vi "HTS_WAIT_FOR_READY.vi"(8 "Error IN":errorcluster, 10 "Polling time(ms)":u32=100, 11 "VISA resource IN":refnum<visa-resource-name>="COM1") -> (0 "Error OUT":errorcluster, 1 "READY?":bool=TRUE, 2 "RESPONSE":string[](array[string])=["SYSTEM STATUS: ", "0x0", "2 PUMPS", "PUMP_1 STATUS: ", "0x60", "PUMP_2 STATUS: ", "0x60", "AXIS X STATUS: ", "0x9", "AXIS Y STATUS: ", "0x9", "AXIS P STATUS: ", "0x9", "AXIS Z STATUS: ", "0x9", "NO ERROR, READY", ">"], 3 "VISA resource OUT":refnum<visa-resource-name>="HTS")   [LabVIEW 2013]
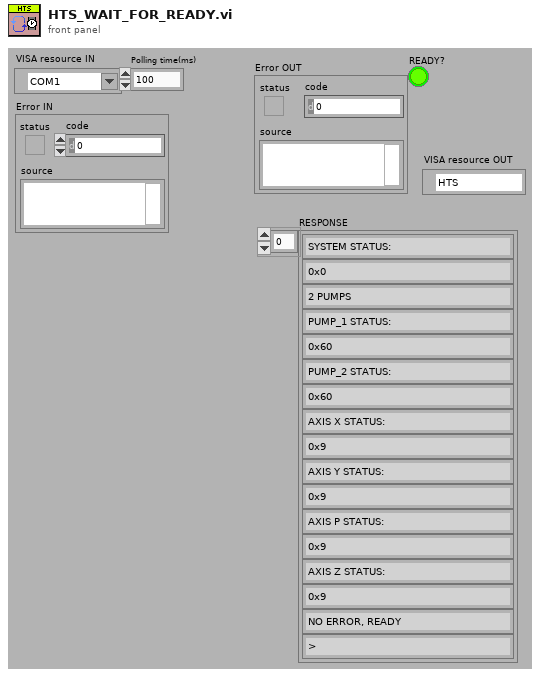
[diagram p1: front panel]
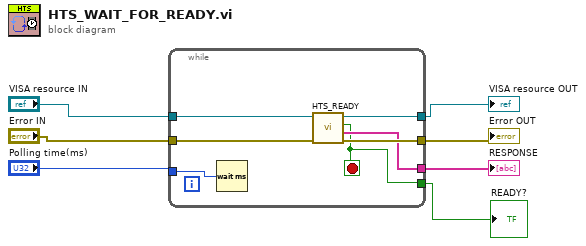
[diagram p0: block diagram]
diagram:
  n1 = while {
    tunnel: "Error IN" -> [w14]
    tunnel: "VISA resource IN" -> [w13]
    tunnel: [w12] -> w5
    tunnel: [w11] -> w4
    tunnel: "Polling time(ms)" -> [w10]
    tunnel: [w9] -> w2
    tunnel: [w8] -> w1
    stop <- w8 stop-if-true
    n2 = Wait (ms)(milliseconds to wait=w10) -> ()  [unwired: 1 out]
    n3 = call "HTS_READY.vi"("Error IN"=w14, "VISA resource IN"=w13) -> ("Error OUT"=w11:errorcluster, "RESPONSE"=w9:string[], "READY?"=w8:bool, "VISA resource OUT"=w12:refnum<visa-resource-name>)  [unwired: 6 out]
  }
  "VISA resource OUT" <- w5
  "Error OUT" <- w4
  "RESPONSE" <- w2
  "READY?" <- w1
